vi "usrp get tx stream.vi"(8 "error in (no error)":errorcluster, 9 "h_out":u64, 10 "stream_args 2":T2, 11 "h":u64) -> (0 "error out":errorcluster, 1 "h_out 2":u64, 2 "stream_args 3":T2, 3 "h 2":u64, 4 "function return":u32(ring))   [LabVIEW 2024, in "uhd.lvlib"]
doc: "UHD_API uhd_error uhd_usrp_get_tx_stream(\n uhd_usrp_handle h, uhd_stream_args_t* stream_args, uhd_tx_streamer_handle h_out);"
uses:
  uhd.lvlib
  uhd.dll
panel:
  in  "stream_args 4":T1
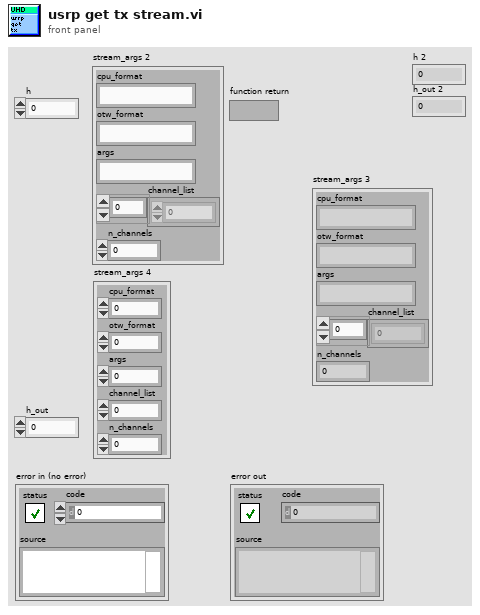
[diagram p1: front panel]
types:
  T1 = cluster{"cpu_format":u64, "otw_format":u64, "args":u64, "channel_list":u64, "n_channels":i32}
  T2 = cluster{"cpu_format":string, "otw_format":string, "args":string, "channel_list":u64[], "n_channels":u64}
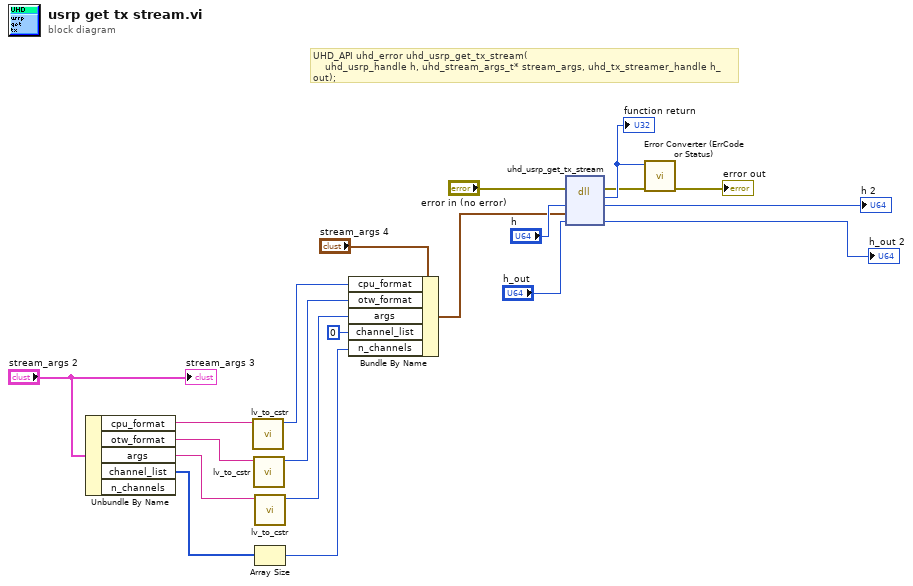
[diagram p0: block diagram]
diagram:
  # "UHD_API uhd_error uhd_usrp_get_tx_stream(\n    uhd_usrp_handle h, uhd_stream_args_t* stream_args, uhd_tx_streamer_handle h_out);"
  n1 = Unbundle By Name("stream_args 2") -> ("cpu_format"=w12:string, "otw_format"=w11:string, "args"=w10:string, "channel_list"=w13:u64[])  [unwired: 1 out]
  n2 = call "lv_to_cstr.vi"("labview string"=w12) -> ("C string"=w8:u64)  [unwired: 9 in, 1 out]
  n3 = call "lv_to_cstr.vi"("labview string"=w11) -> ("C string"=w7:u64)  [unwired: 9 in, 1 out]
  n4 = call "lv_to_cstr.vi"("labview string"=w10) -> ("C string"=w6:u64)  [unwired: 9 in, 1 out]
  n5 = Array Size(array=w13) -> (size(s)=w4:i32)
  n6 = Bundle By Name(cluster="stream_args 4", "cpu_format"=w8, "otw_format"=w7, "args"=w6, "channel_list"=u64 0, "n_channels"=w4) -> (w3:T1)
  n7 = dll-call lib="uhd.dll" fn="uhd_usrp_get_tx_stream"(error in="error in (no error)", "h"="h", "stream_args"=w3, "h_out"="h_out") -> (error out=w16:errorcluster, "return type"=w20:u32, "h"=→"h 2":u64, "h_out"=→"h_out 2":u64)  [unwired: 3 in, 1 out]
  "function return" <- w20
  n8 = call "Error Converter (ErrCode or Status).vi"("error in (no error)"=w16, "error code"=w20) -> ("error out"=→"error out":errorcluster)  [unwired: 9 in]
  "stream_args 3" <- "stream_args 2"
